vi "readValue.vi"(8 "error in (no error)":errorcluster, 9 "id":T2=1, 10 "CoolerQuery":T3, 11 "CoolerControler in":refnum<class "CoolerControler.lvclass">) -> (0 "error out":errorcluster, 1 "response out":T1, 2 "validChecksum":bool, 3 "CoolerControler out":refnum<class "CoolerControler.lvclass">)   [LabVIEW 2016, in "CoolerControler.lvclass"]
uses:
  CoolerControler.lvclass
  typedefs/CoolerQuery.ctl
  typedefs/CoolerId.ctl
  typedefs/response.ctl
  SerialCommand/CoolerSerialCommand.lvclass
  typedefs/typeOfCommand.ctl
  CoolerControler.lvclass/CoolerControler.ctl
  common_serial_tcpextended/Communicator/Communicator.lvclass
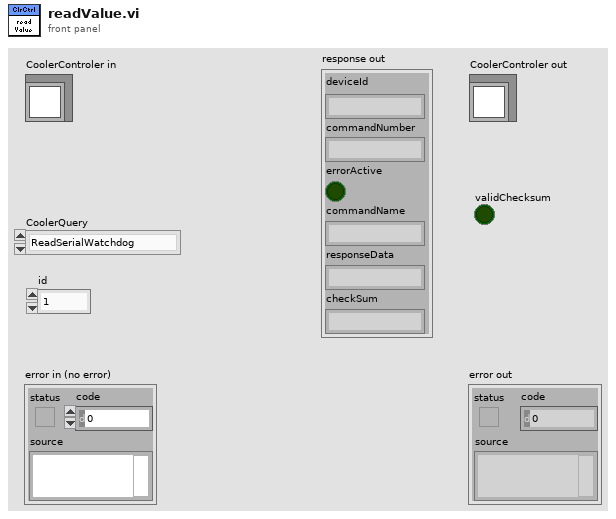
[diagram p1: front panel]
types:
  T1 = typedef "response.ctl" = cluster{"deviceId":string, "commandNumber":string, "errorActive":bool, "commandName":string, "responseData":string, "checkSum":string}
  T2 = typedef "CoolerId.ctl" = u16
  T3 = typedef "CoolerQuery.ctl" = enum16{"ReadSerialWatchdog", "ReadControlSensor", "ReadSetTemperature", "ReadSupplyTemperature", "ReadExternalRTD", "ReadExternalThermistor", "ReadReturnTemperature", "ReadAmbientTemperature", "ReadProcessFlow", "ReadTECBank1Current", "ReadTECBank2Current", "ReadTEDriveLevel", "ReadAlarmStateLevel1", "ReadAlarmStateLevel21", "ReadAlarmStateLevel22", "ReadWarningStateLevel1", "ReadHighSupplyTempWarning", "ReadLowSupplyTempWarning", "ReadHighAmbientTempWarning", "ReadLowAmbientTempWarning", "ReadLowProcessFlowWarning", "ReadHighSupplyTempAlarm", "ReadLowSupplyTempAlarm", "ReadHighAmbientTempAlarm", "ReadLowAmbientTempAlarm", "ReadLowProcessFlowAlarm", "ReadPWMandRelayStatus", "ReadPIDStatus", "ReadUnitUpTime", "ReadFan1Speed", "ReadFan2Speed", "ReadFan3Speed", "ReadFan4Speed"}
  T4 = typedef "typeOfCommand.ctl" = enum16{"command", "response"}
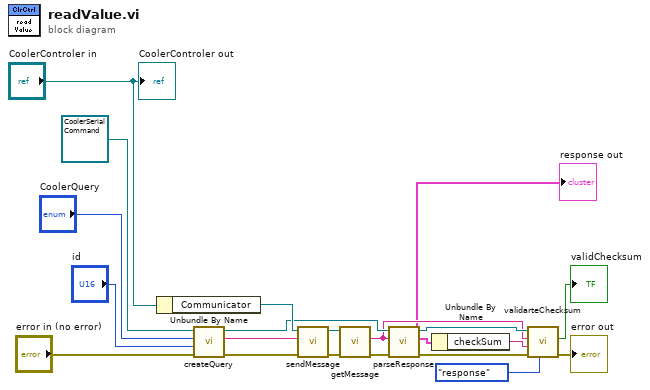
[diagram p0: block diagram]
diagram:
  n1 = Unbundle By Name("CoolerControler in") -> ("Communicator"=w15:refnum<class "Communicator.lvclass">)
  n2 = call "createQuery.vi"("error in (no error)"="error in (no error)", "id"="id", "CoolerQuery"="CoolerQuery", "CoolerSerialCommand in"=refnum<class "CoolerSerialCommand.lvclass"> refnum ("CoolerSerialCommand.lvclass")) -> ("error out"=w12:errorcluster, "SerialQueryStr"=w13:string, "CoolerSerialCommand out"=w10:refnum<class "CoolerSerialCommand.lvclass">)  [unwired: 5 in]
  n3 = call-dynamic "sendMessage.vi"("error in (no error)"=w12, "message"=w13, "Communicator in"=w15) -> ("error out"=w11:errorcluster, "Communicator out"=w14:refnum<class "Communicator.lvclass">)  [unwired: 7 in]
  n4 = call-dynamic "getMessage.vi"("error in (no error)"=w11, "Communicator in"=w14) -> ("error out"=w9:errorcluster, "String"=w4:string)  [unwired: 7 in, 1 out]
  n5 = call "parseResponse.vi"("error in (no error)"=w9, "response in"=w4, "CoolerSerialCommand in"=w10) -> ("error out"=w7:errorcluster, "response out"=w3:T1, "CoolerSerialCommand out"=w8:refnum<class "CoolerSerialCommand.lvclass">)  [unwired: 6 in]
  "response out" <- w3
  n6 = Unbundle By Name(w3) -> ("checkSum"=w2:string)
  n7 = call "validarteChecksum.vi"("messageType"=typeOfCommand."response", "error in (no error)"=w7, "checkSum"=w2, "response"=w4, "CoolerSerialCommand in"=w8) -> ("error out"=→"error out":errorcluster, "validChecksum"=→"validChecksum":bool)  [unwired: 4 in, 1 out]
  "CoolerControler out" <- "CoolerControler in"
